vi "SbigCloseSynchronization.vi"(3 "Queue in":T2, 7 "Notifiers in":T1[](array[typedef]), 9 "error in (no error)":errorcluster) -> (6 "error out (no error)":errorcluster caption="error out")   [LabVIEW 2009]
uses:
  Controls/SbigCommandQueue.ctl
  Controls/SbigCommand.ctl
  Controls/SbigStatusNotifier.ctl
  Controls/SbigStatus.ctl
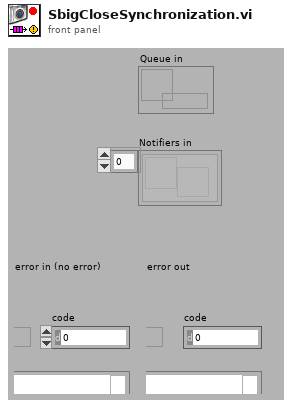
[diagram p1: front panel]
types:
  T1 = typedef "SbigStatusNotifier.ctl" = refnum<notifier>
  T2 = typedef "SbigCommandQueue.ctl" = refnum<queue>
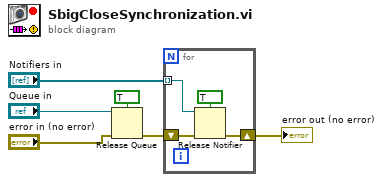
[diagram p0: block diagram]
diagram:
  n1 = Release Queue(queue="Queue in", force destroy? (F)=TRUE ("forcer la destruction ? (F)"), error in (no error)="error in (no error)") -> (error out=w5:errorcluster)  [unwired: 2 out]
  n2 = for {
    tunnel: "Notifiers in" -> [w9] mode=indexing
    shift-right: [w7] -> w6
    shift-left: w5 -> [w10]
    n3 = Release Notifier(notifier=w9, force destroy? (F)=TRUE ("forcer la destruction ? (F)"), error in (no error)=w10) -> (error out=w7:errorcluster)  [unwired: 2 out]
  }
  "error out (no error)" <- w6
